vi "Polling Stop Core.vi"(8 "Error In":errorcluster, 11 "BNT_DAQmx-MCSV-DOPWM in":refnum<class "BNT_DAQmx-MCSV-DOPWM.lvclass">) -> (0 "Error Out":errorcluster, 3 "BNT_DAQmx-MCSV-DOPWM out":refnum<class "BNT_DAQmx-MCSV-DOPWM.lvclass">)   [LabVIEW 2021, in "BNT_DAQmx.lvlib" / "BNT_DAQmx-MCSV-DOPWM.lvclass"]
doc: "Implement your code to stop polling here."
uses:
  BNT_DAQmx-MCSV-DOPWM.lvclass
  C:/Users/Holger/Documents/LVP/BNT/EQCR/Packages/BNT_DAQmx/BNT_DAQmx-MCSV/BNT_DAQmx-MCSV.lvclass
  BNT_DAQmx-MCSV/BNT_DAQmx-MCSV.lvclass/BNT_DAQmx-MCSV.ctl
  BNT_DAQmx-MCSV/BNT_DAQmx-MCSV.lvclass
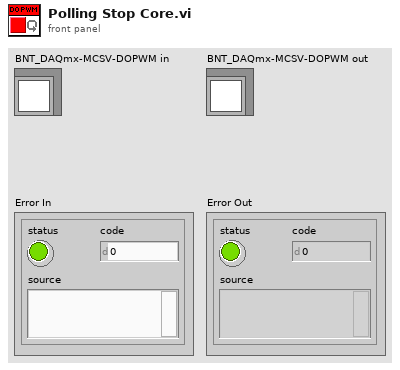
[diagram p1: front panel]
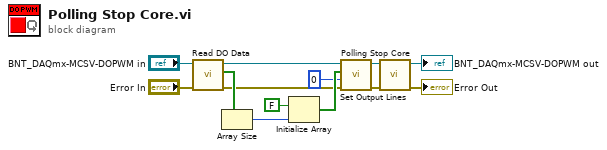
[diagram p0: block diagram]
diagram:
  n1 = call "Read DO Data.vi"("error in (no error)"="Error In", "BNT_DAQmx-MCSV in"="BNT_DAQmx-MCSV-DOPWM in") -> ("error out"=w1:errorcluster, "DO Data"=w5:bool[], "BNT_DAQmx-MCSV out"=w3:refnum<class "BNT_DAQmx-MCSV-DOPWM.lvclass">)  [unwired: 7 in]
  n2 = Array Size(array=w5) -> (size(s)=w8:i32)
  n3 = Initialize Array(FALSE, w8) -> (w7:bool[])
  n4 = call "Set Output Lines.vi"("Error In"=w1, "Start Index"=0, "DO Lines"=w7, "BNT_DAQmx-MCSV in"=w3) -> ("Error Out"=w10:errorcluster, "BNT_DAQmx-MCSV out"=w11:refnum<class "BNT_DAQmx-MCSV-DOPWM.lvclass">)  [unwired: 6 in]
  n5 = call-parent "Polling Stop Core.vi"("Error In"=w10, "CSPP_BaseActor in"=w11) -> ("Error Out"=→"Error Out":errorcluster, "CSPP_BaseActor out"=→"BNT_DAQmx-MCSV-DOPWM out":refnum<class "BNT_DAQmx-MCSV-DOPWM.lvclass">)  [unwired: 8 in]
